vi "KLegend Test.vi"() -> ()   [LabVIEW 2020]
uses:
  KLegend/KLegend.xctl
  Math VIs/LinSpace (x0-dx-npts).vi
  <vilib>/Analysis/NI_AALBase.lvlib
panel:
  in  "stop":bool
  out "KLegend":i32(xcontrol)
  out "XY Graph":T1(graph)
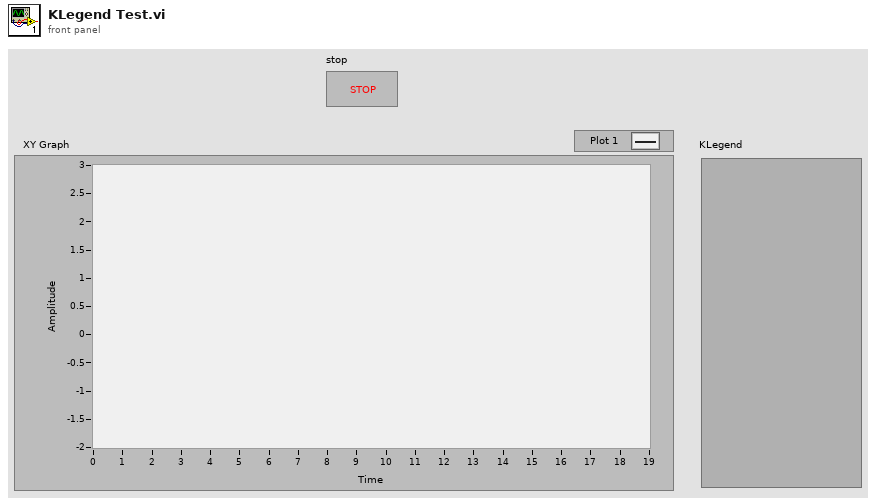
[diagram p1: front panel]
types:
  T1 = cluster{"Array":dbl[], "Gaussian noise pattern":dbl[]}[]
  T2 = enum16{"User", "Prism", "Kelly", "Dark2", "Sequential", "Hue"}
  T3 = cluster{"Array":dbl[], "Gaussian noise pattern":dbl[]}
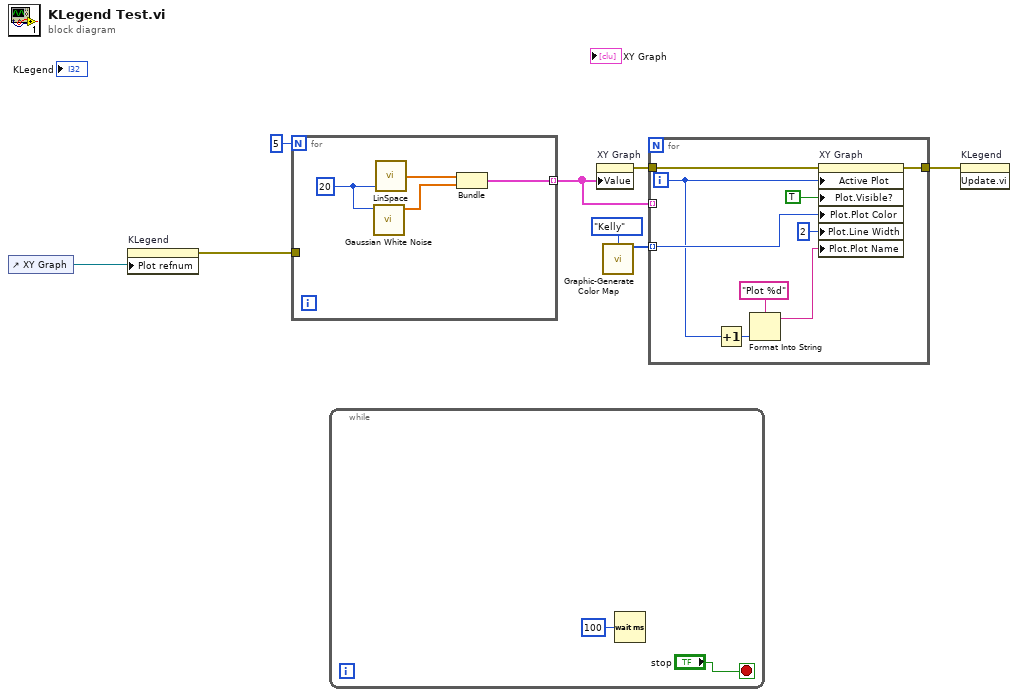
[diagram p0: block diagram]
diagram:
  n1 = control-ref of="XY Graph"() -> (w8:refnum<vi>)
  n2 = property on="KLegend" class="KLegend (strict)"("Plot refnum"=w8) -> (error out=w6:errorcluster)  [unwired: 2 in, 1 out]
  n3 = for {
    N: 5 -> [_]
    tunnel: [w9] -> w4 mode=indexing
    tunnel: w6 -> [_]
    w12 = 20 ("samples")
    n4 = call <vilib>:"Gaussian White Noise.vi"("samples"=w12) -> ("Gaussian noise pattern"=w10:dbl[])  [unwired: 9 in, 1 out]
    n5 = call-poly "LinSpace.vi"("npts"=w12) -> ("Array"=w11:dbl[])  [unwired: 3 in, 1 out]
    n6 = Bundle("Array"=w11, "Gaussian noise pattern"=w10) -> (w9:T3)  [unwired: 1 in]
  }
  n7 = while {
    stop <- "stop" stop-if-true
    n8 = Wait (ms)(milliseconds to wait=u32 100) -> ()  [unwired: 1 out]
  }
  n9 = property on="XY Graph" class="XYGraph (strict)"("Value"=w4) -> (error out=w5:errorcluster)  [unwired: 2 in, 1 out]
  n10 = call "Graphic-Generate Color Map.vi"("Map"=T2."Kelly") -> ("Colors"=w1:u32[])  [unwired: 14 in]
  n11 = for {
    tunnel: w5 -> [w23]
    tunnel: w4 -> [_] mode=indexing
    tunnel: [w21] -> w3
    tunnel: w1 -> [w20] mode=indexing
    i -> [w15]
    n12 = Increment(x=w15) -> (x+1=w16:i32)
    n13 = Format Into String(format string="Plot %d", w16) -> (resulting string=w18:string)  [unwired: 2 in, 1 out]
    n14 = property on="XY Graph" class="XYGraph (strict)"(error in=w23, "Active Plot"=w15, "Plot.Visible?"=TRUE ("Plot.Visible"), "Plot.Plot Color"=w20, "Plot.Line Width"=u8 2, "Plot.Plot Name"=w18) -> (error out=w21:errorcluster)  [unwired: 1 in, 1 out]
  }
  n15 = invoke on="KLegend" class="KLegend (strict)" method="Update.vi"(error in=w3) -> ()  [unwired: 2 in, 3 out]
